vi "LV2 - Mark10MonitorQueue.vi"(7 "Enum":enum16{"Set", "Get"}(ring)=enum."Get", 11 "Mark10Monitor":refnum<queue>) -> (3 "Mark10Monitor out":refnum<queue>)   [LabVIEW 2019, in "Mark 10 TSTM-DC.lvlib" / "Mark 10 Event Monitor.lvlib"]
uses:
  Mark 10 Event Monitor.lvlib
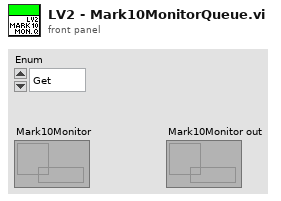
[diagram p1: front panel]
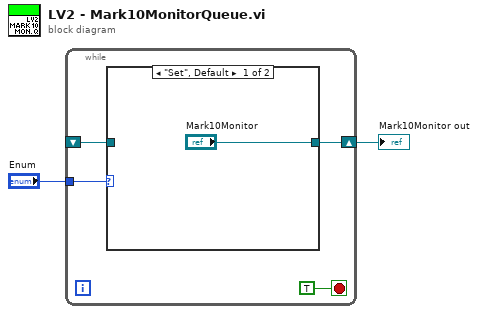
[diagram p0: block diagram]
diagram:
  n1 = while {
    shift-right: [w6] -> w1
    shift-left: _ -> [w5]
    tunnel: "Enum" -> [w4]
    stop <- TRUE stop-if-true
    n2 = case shown="\"Set\", Default" w4 {
      tunnel: ["Mark10Monitor" w8] -> w6
      tunnel: w5 -> [_ w8]
      frame "Set", Default {
      }
      frame "Get" {
      }
    }
  }
  "Mark10Monitor out" <- w1
